vi "Determine Change List.vi"(8 "error in (no error)":errorcluster, 10 "Old Cluster":refnum<k21>="NI_Support_20250912", 11 "New Cluster":refnum<k21>="NI_Support_20250912_New") -> (0 "error out":errorcluster, 1 "Changed":T2[](array[typedef]), 2 "Missing":T1[](array[typedef]), 3 "New":T1[](array[typedef]))   [LabVIEW 2025, in "Protection and Counter Addon System Explorer.lvlib"]
uses:
  Protection and Counter Addon System Explorer.lvlib
  Types/Related CAN Frames No VS.ctl
  Types/Base Frame Info_NoVS.ctl
  <resource>/objmgr/xnet.rc
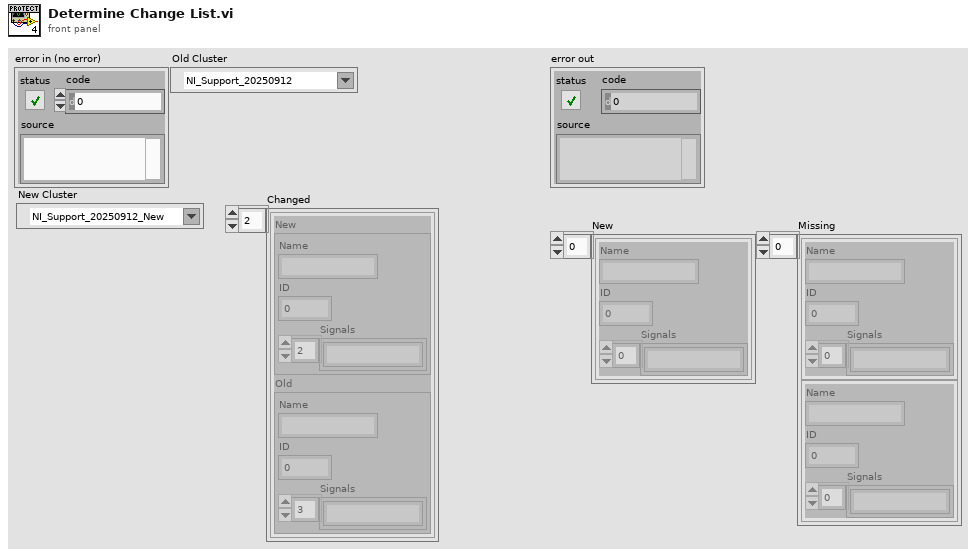
[diagram p1: front panel]
types:
  T1 = typedef "Protection and Counter Addon System Explorer.lvlib/Base Frame Info_NoVS.ctl" = cluster{"Name":string, "ID":u32, "Signals":string[]}
  T2 = typedef "Protection and Counter Addon System Explorer.lvlib/Related CAN Frames No VS.ctl" = cluster{"New":T1, "Old":T1}
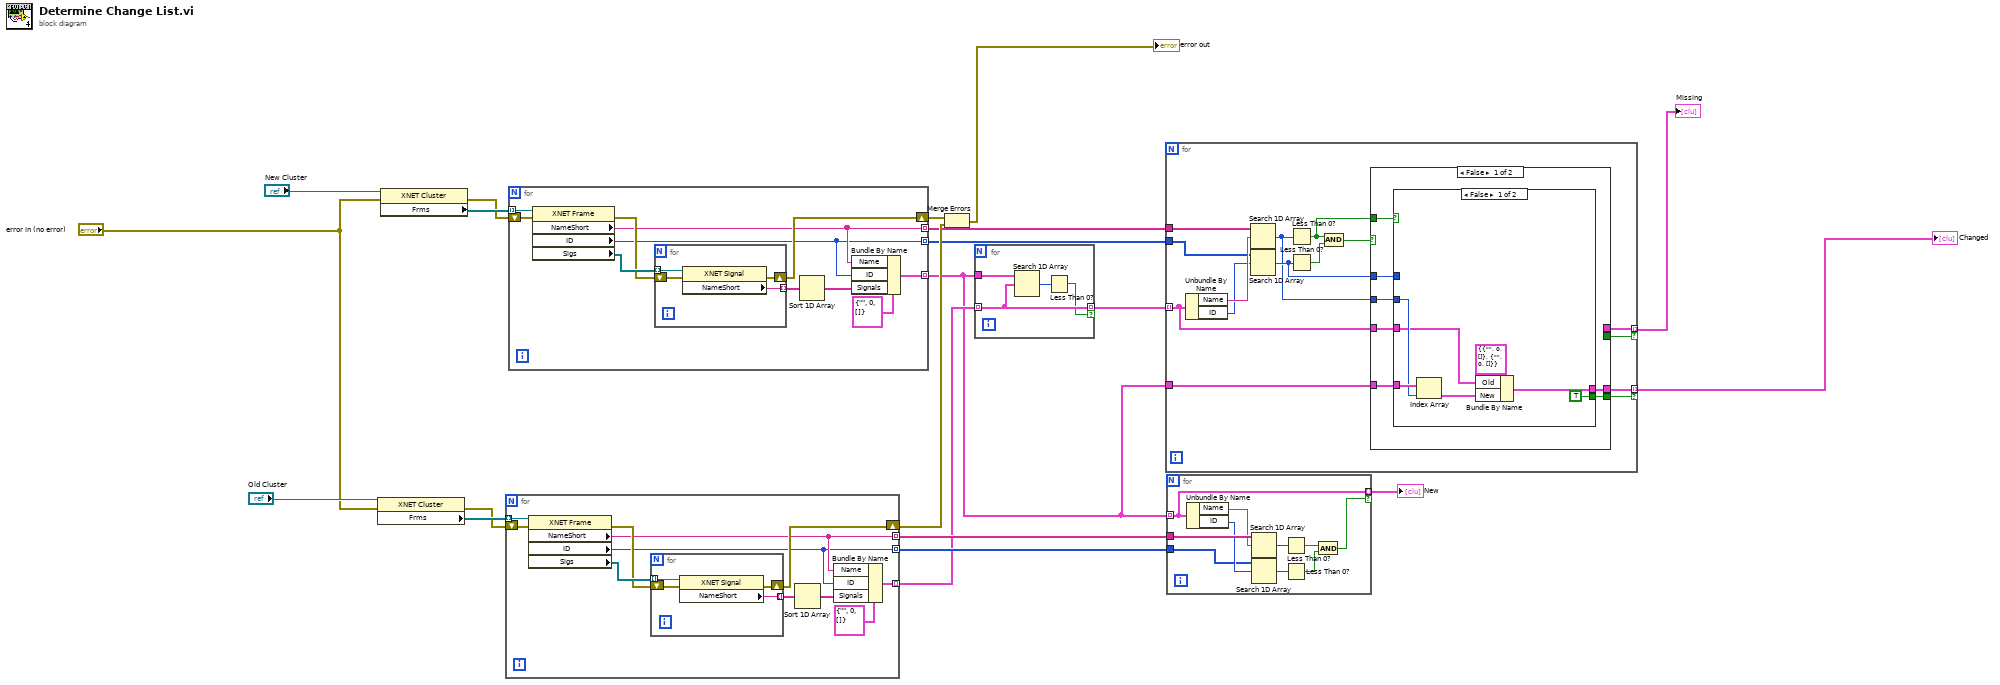
[diagram p0: block diagram]
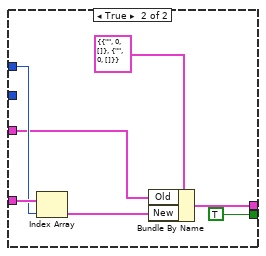
[diagram p2: hidden frame]
diagram:
  n1 = property class="XNET Cluster"(reference="Old Cluster", error in="error in (no error)") -> (error out=w16:errorcluster, "Frms"=w17:refnum<k21>[])  [unwired: 1 out]
  n2 = property class="XNET Cluster"(reference="New Cluster", error in="error in (no error)") -> (error out=w18:errorcluster, "Frms"=w19:refnum<k21>[])  [unwired: 1 out]
  n3 = for {
    tunnel: w17 -> [w31] mode=indexing
    shift-right: [w23] -> w12
    shift-left: w16 -> [w30]
    tunnel: [w27] -> w7 mode=indexing
    tunnel: [w22] -> w10 mode=indexing
    tunnel: [w21] -> w9 mode=indexing
    n4 = property class="XNET Frame"(reference=w31, error in=w30) -> (error out=w24:errorcluster, "NameShort"=w22:string, "ID"=w21:u32, "Sigs"=w29:refnum<k21>[])  [unwired: 1 out]
    n5 = for {
      tunnel: w29 -> [w35] mode=indexing
      shift-right: [w33] -> w23
      shift-left: w24 -> [w34]
      tunnel: [w32] -> w28 mode=indexing
      n6 = property class="XNET Signal"(reference=w35, error in=w34) -> (error out=w33:errorcluster, "NameShort"=w32:string)  [unwired: 1 out]
    }
    n7 = Sort 1D Array(array=w28) -> (sorted array=w25:string[])
    n8 = Bundle By Name(cluster=T1 {"Name"="", "ID"=0, "Signals"=[]}, "Name"=w22, "ID"=w21, "Signals"=w25) -> (w27:T1)
  }
  n9 = for {
    tunnel: w19 -> [w46] mode=indexing
    shift-right: [w38] -> w13
    shift-left: w18 -> [w45]
    tunnel: [w42] -> w2 mode=indexing
    tunnel: [w37] -> w4 mode=indexing
    tunnel: [w36] -> w3 mode=indexing
    n10 = property class="XNET Frame"(reference=w46, error in=w45) -> (error out=w39:errorcluster, "NameShort"=w37:string, "ID"=w36:u32, "Sigs"=w44:refnum<k21>[])  [unwired: 1 out]
    n11 = for {
      tunnel: w44 -> [w50] mode=indexing
      shift-right: [w48] -> w38
      shift-left: w39 -> [w49]
      tunnel: [w47] -> w43 mode=indexing
      n12 = property class="XNET Signal"(reference=w50, error in=w49) -> (error out=w48:errorcluster, "NameShort"=w47:string)  [unwired: 1 out]
    }
    n13 = Sort 1D Array(array=w43) -> (sorted array=w40:string[])
    n14 = Bundle By Name(cluster=T1 {"Name"="", "ID"=0, "Signals"=[]}, "Name"=w37, "ID"=w36, "Signals"=w40) -> (w42:T1)
  }
  n15 = Merge Errors(w13, w12) -> (→"error out":errorcluster)
  n16 = for {
    tunnel: w2 -> [w54]
    tunnel: w7 -> [w52] mode=indexing
    tunnel: [w52] -> w5 mode=indexing if=w51
    n17 = Search 1D Array(1D array=w54, element=w52) -> (index of element=w53:i32)  [unwired: 1 in]
    n18 = Less Than 0?(x=w53) -> (x < 0?=w51:bool)
  }
  n19 = for {
    tunnel: w5 -> [w63] mode=indexing
    tunnel: w4 -> [w69]
    tunnel: w3 -> [w66]
    tunnel: [w62] -> w6 mode=indexing if=w61
    tunnel: w2 -> [w59]
    tunnel: [w56] -> w1 mode=indexing if=w55
    n20 = Unbundle By Name(w63) -> ("Name"=w68:string, "ID"=w67:u32)
    n21 = Search 1D Array(1D array=w69, element=w68) -> (index of element=w57:i32)  [unwired: 1 in]
    n22 = Search 1D Array(1D array=w66, element=w67) -> (index of element=w58:i32)  [unwired: 1 in]
    n23 = Less Than 0?(x=w57) -> (x < 0?=w60:bool)
    n24 = Less Than 0?(x=w58) -> (x < 0?=w65:bool)
    n25 = Compound Arithmetic op=AND(w60, w65) -> (w64:bool)
    n26 = case shown="False" w64 {
      selector: w64 -> [_ w91]
      tunnel: w63 -> [w72 w92]
      tunnel: [_ w92] -> w62
      tunnel: [_ w91] -> w61
      tunnel: w60 -> [w76 _]
      tunnel: w59 -> [w75 _]
      tunnel: w58 -> [w74 _]
      tunnel: w57 -> [w73 _]
      tunnel: [w71 _] -> w56
      tunnel: [w70 _] -> w55
      frame False {
        n27 = case shown="False" w76 {
          tunnel: w75 -> [w83 w90]
          tunnel: w74 -> [_ w89]
          tunnel: w73 -> [w82 _]
          tunnel: w72 -> [w78 w86]
          tunnel: [w77 w85] -> w71
          tunnel: [TRUE TRUE] -> w70
          frame False {
            n28 = Index Array(array=w83, index=w82) -> (element=w79:T1)
            n29 = Bundle By Name(cluster=T2 {"New"={"Name"="", "ID"=0, "Signals"=[]}, "Old"={"Name"="", "ID"=0, "Signals"=[]}}, "Old"=w78, "New"=w79) -> (w77:T2)
          }
          frame True {
            n30 = Index Array(array=w90, index=w89) -> (element=w87:T1)
            n31 = Bundle By Name(cluster=T2 {"New"={"Name"="", "ID"=0, "Signals"=[]}, "Old"={"Name"="", "ID"=0, "Signals"=[]}}, "Old"=w86, "New"=w87) -> (w85:T2)
          }
        }
      }
      frame True {
      }
    }
  }
  "Changed" <- w1
  "Missing" <- w6
  n32 = for {
    tunnel: w2 -> [w94] mode=indexing
    tunnel: w10 -> [w102]
    tunnel: w9 -> [w99]
    tunnel: [w94] -> w8 mode=indexing if=w93
    n33 = Unbundle By Name(w94) -> ("Name"=w101:string, "ID"=w100:u32)
    n34 = Search 1D Array(1D array=w102, element=w101) -> (index of element=w98:i32)  [unwired: 1 in]
    n35 = Search 1D Array(1D array=w99, element=w100) -> (index of element=w97:i32)  [unwired: 1 in]
    n36 = Less Than 0?(x=w98) -> (x < 0?=w96:bool)
    n37 = Less Than 0?(x=w97) -> (x < 0?=w95:bool)
    n38 = Compound Arithmetic op=AND(w96, w95) -> (w93:bool)
  }
  "New" <- w8
